vi "day1.vi"() -> ()   [LabVIEW 2025]
panel:
  out "Array":i32[](array[numeric])
  in  "Test":bool
  out "result":i32
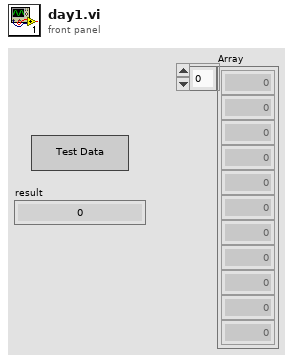
[diagram p1: front panel]
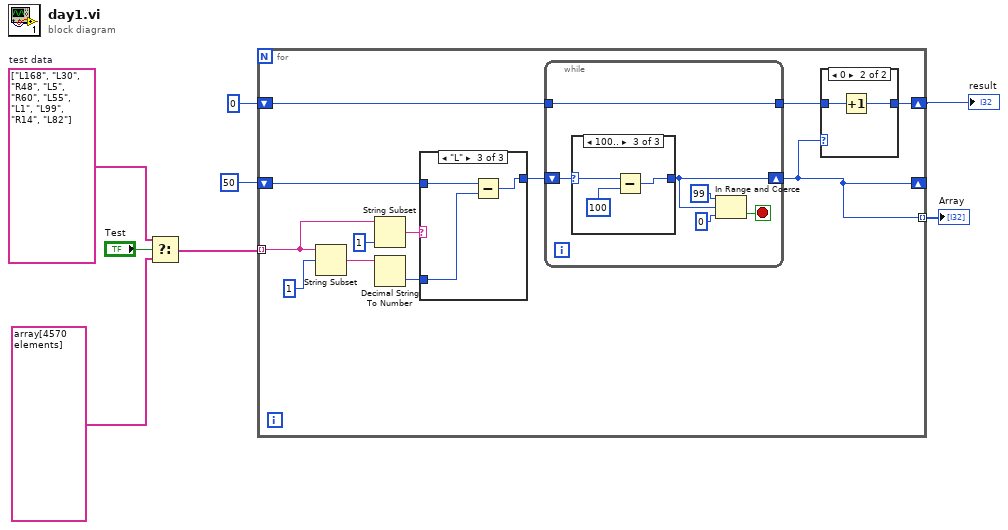
[diagram p0: block diagram]
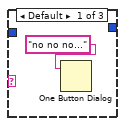
[diagram p2: hidden frame]
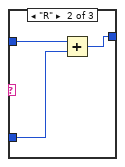
[diagram p3: hidden frame]
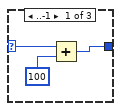
[diagram p4: hidden frame]
diagram:
  w5 = string[] ["L168", "L30", "R48", "L5", "R60", "L55", "L1", "L99", "R14", "L82"]  # test data
  n1 = Select(t=w5, s="Test", f=string[] array[4570 elements]) -> (s? t:f=w6:string[])
  n2 = for {
    tunnel: w6 -> [w16] mode=indexing
    shift-right: [w11] -> _
    shift-left: 50 -> [w18]
    shift-right: [w17] -> w7
    shift-left: 0 -> [w9]
    tunnel: [w11] -> w3 mode=indexing
    n3 = String Subset(string=w16, offset (0)=1) -> (substring=w19:string)  [unwired: 1 in]
    n4 = String Subset(string=w16, length (rest)=1 ("length (rest)")) -> (substring=w15:string)  [unwired: 1 in]
    n5 = Decimal String To Number(string=w19) -> (number=w13:i32)  [unwired: 2 in, 1 out]
    n6 = case shown="\"L\"" w15 {
      tunnel: w13 -> [_ w24 w27]
      tunnel: [_ w23 w26] -> w12
      tunnel: w18 -> [_ w22 w25]
      frame Default {
        n7 = One Button Dialog(message="no no no...") -> ()  [unwired: 1 in, 1 out]
      }
      frame "R" {
        n8 = Add(x=w22, y=w24) -> (x+y=w23:i32)
      }
      frame "L" {
        n9 = Subtract(x=w25, y=w27) -> (x-y=w26:i32)
      }
    }
    n10 = while {
      shift-right: [w31] -> w11
      shift-left: w12 -> [w33]
      tunnel: [w28] -> w10
      tunnel: w9 -> [w28]
      stop <- w32 stop-if-true
      n11 = case shown="100.." w33 {
        selector: w33 -> [w36 w37 w40]
        tunnel: [w35 w37 w39] -> w31
        frame ..-1 {
          n12 = Add(x=w36, y=100) -> (x+y=w35:i32)
        }
        frame 0, Default {
        }
        frame 100.. {
          n13 = Subtract(x=w40, y=100) -> (x-y=w39:i32)
        }
      }
      n14 = In Range and Coerce(upper limit=99, x=w31, lower limit=0) -> (In Range?=w32:bool)  [unwired: 1 out]
    }
    n15 = case shown="0" w11 {
      tunnel: w10 -> [w41 w43]
      tunnel: [w41 w42] -> w17
      frame Default {
      }
      frame 0 {
        n16 = Increment(x=w43) -> (x+1=w42:i32)
      }
    }
  }
  "result" <- w7
  "Array" <- w3
